vi "Call.vi"(0 "WAMP Client in":refnum<class "WAMP Client.lvclass">, 5 "error in (no error)":errorcluster, 7 "Topic URI":string, 9 "Arguments":variant[](array[variant]), 11 "ArgumentsKw":string) -> (4 "WAMP Client out":refnum<class "WAMP Client.lvclass">, 6 "error out":errorcluster, 8 "Success?":bool, 10 "Arguments Payload":string[](array[string]), 15 "ArgumentKw Payload":string)   [LabVIEW 2020, in "WAMP Client.lvclass"]
uses:
  <userlib>/lvwamp/WAMP Client/WAMP Client.lvclass
  <userlib>/lvwamp/WAMP Client/TypeDef/Internal Message Type.ctl
  <userlib>/lvwamp/WAMP Client/TypeDef/CALL Request Data.ctl
  <userlib>/lvwamp/WAMP Client/TypeDef/RESULT Payload.ctl
  <vilib>/Utility/error.llb/Error Cluster From Error Code.vi
  <vilib>/ErrorRing/Error Ring.xnode
panel:
  in  "Numeric":i32=500
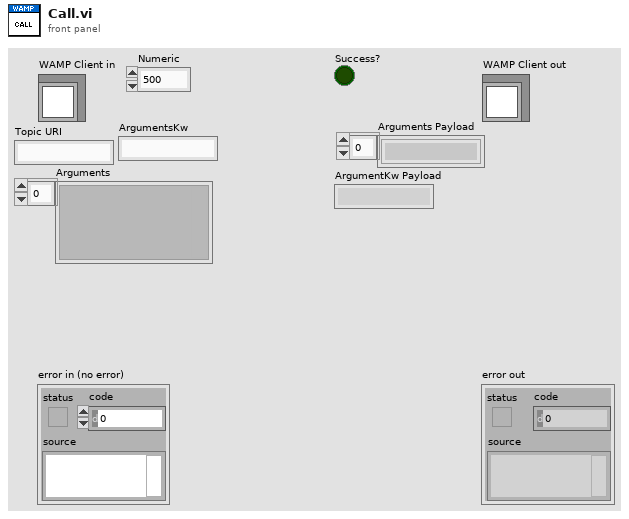
[diagram p1: front panel]
types:
  T1 = typedef "WAMP Client.lvclass/RESULT Payload.ctl" = cluster{"Arguments Payload":string[], "ArgumentKw Payload":string, "Topic":string, "Success?":bool, "Error":errorcluster}
  T2 = typedef "WAMP Client.lvclass/CALL Request Data.ctl" = cluster{"Topic URI":string, "Arguments":variant[], "ArgumentsKw":string, "Result Received":refnum<user-event>}
  T3 = typedef "WAMP Client.lvclass/Internal Message Type.ctl" = enum16{"Subscribe", "Handle Subscribed", "Handle Event", "Unsubscribe", "Handle Unsubscribed", "Publish", "Handled Published", "Goodbye", "Handle Goodbye", "Call", "Handle Result"}
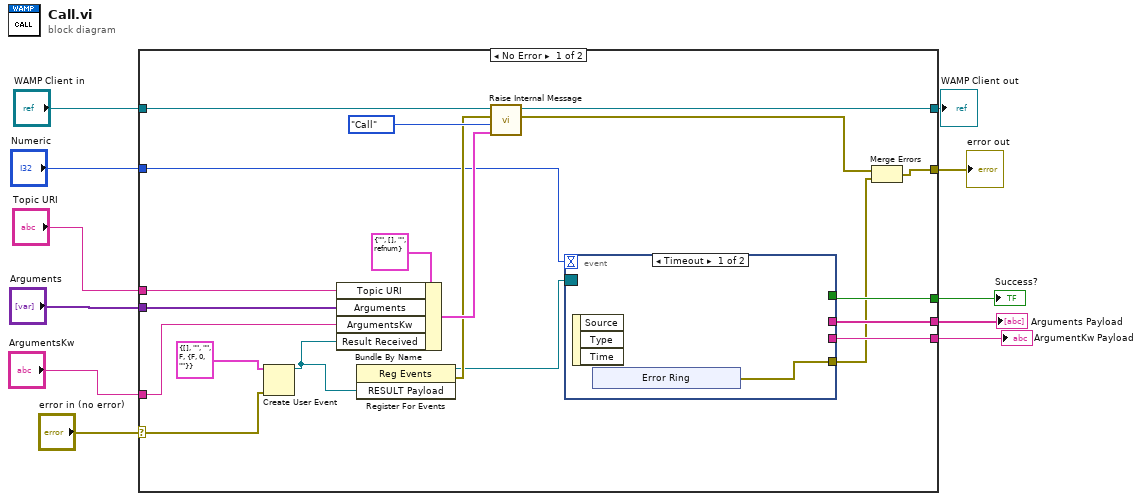
[diagram p0: block diagram]
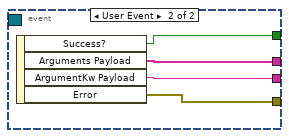
[diagram p2: hidden frame]
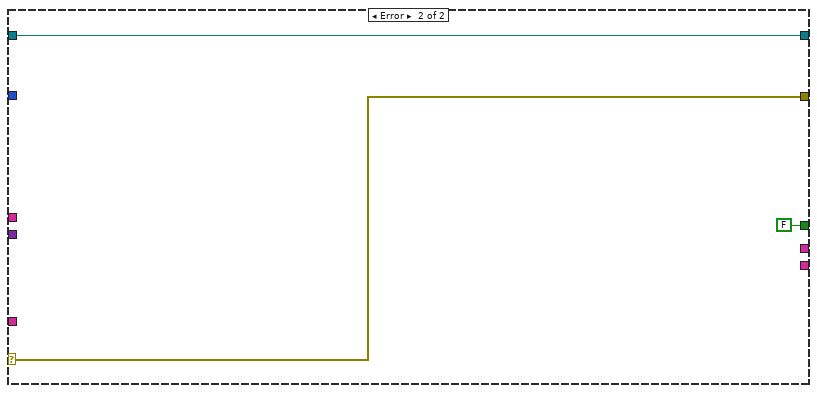
[diagram p3: hidden frame]
diagram:
  n1 = case shown="No Error" "error in (no error)" {
    selector: "error in (no error)" -> [w22 w44]
    tunnel: [w12 w44] -> w10
    tunnel: [w30 w43] -> w8
    tunnel: "WAMP Client in" -> [w31 w43]
    tunnel: "Topic URI" -> [w27 _]
    tunnel: "Arguments" -> [w26 _]
    tunnel: "ArgumentsKw" -> [w25 _]
    tunnel: "Numeric" -> [w18 _]
    tunnel: [w17 _] -> w3
    tunnel: [w16 FALSE ("Success?")] -> w2
    tunnel: [w15 _] -> w1
    frame No Error {
      n2 = Create User Event(user event datatype=T1 {"Arguments Payload"=[], "ArgumentKw Payload"="", "Topic"="", "Success?"=FALSE, "Error"={"status"=FALSE, "code"=0, "source"=""}} ("RESULT Payload"), error in=w22) -> (user event=w21:refnum<user-event>)  [unwired: 1 out]
      n3 = Bundle By Name(cluster=T2 {"Topic URI"="", "Arguments"=[], "ArgumentsKw"="", "Result Received"=refnum} ("Call Request"), "Topic URI"=w27, "Arguments"=w26, "ArgumentsKw"=w25, "Result Received"=w21) -> (w24:T2)
      n4 = register-events(w21) -> (reference out=w19:refnum<event-registration>, error out=w20:errorcluster)  [unwired: 2 in]
      n5 = call-dynamic "Raise Internal Message.vi"("Variant"=w24, "Internal Message Type"=Internal_Message_Type."Call", "error in (no error)"=w20, "WAMP Client in"=w31) -> ("error out"=w13:errorcluster, "WAMP Client out"=w30:refnum<class "WAMP Client.lvclass">)  [unwired: 6 in]
      n6 = event shown="[0] Timeout" {
        selector: w19 -> [_ _]
        dyn-events: _ -> [_ _]
        timeout: w18 -> [_ _]
        tunnel: [_ w41] -> w16
        tunnel: [_ w40] -> w17
        tunnel: [_ w39] -> w15
        tunnel: [w32 w38] -> w14
        event Timeout {
          n7 = event-data() -> ()  [unwired: 1 in, 3 out]
          n8 = xnode "Error Ring"() -> ("error out"=w32:errorcluster)
        }
        event User Event {
          n9 = event-data() -> ("Success?"=w41:bool, "Arguments Payload"=w40:string[], "ArgumentKw Payload"=w39:string, "Error"=w38:errorcluster)  [unwired: 1 in]
        }
      }
      n10 = Merge Errors(w13, w14) -> (w12:errorcluster)
    }
    frame Error {
    }
  }
  "error out" <- w10
  "WAMP Client out" <- w8
  "Arguments Payload" <- w3
  "Success?" <- w2
  "ArgumentKw Payload" <- w1
